vi "Read Sample Container.vi"(8 "error in (no error)":errorcluster, 11 "Preparation Line in":refnum<class "Preparation Line.lvclass">) -> (0 "error out":errorcluster, 1 "Sample":refnum<class "Sample.lvclass">, 2 "Container":T1, 3 "Preparation Line out":refnum<class "Preparation Line.lvclass">)   [LabVIEW 2015, in "cRIO-Carbondioxide.lvlib" / "CO2-Actor.lvlib" / "Preparation Line.lvclass"]
uses:
  Preparation Line.lvclass
  subs/Sample/Sample.lvclass
  Controls/Sample Container.ctl
  Preparation Line.lvclass/Preparation Line.ctl
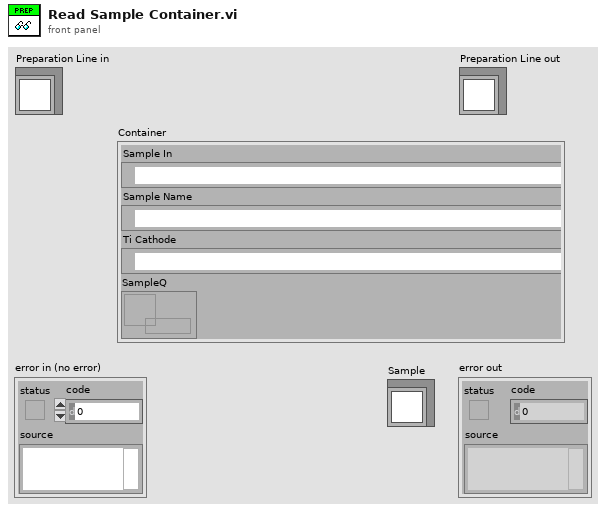
[diagram p1: front panel]
types:
  T1 = typedef "Sample Container.ctl" = cluster{"Sample In":refnum<k21>, "Sample Name":refnum<k21>, "Ti Cathode":refnum<k21>, "SampleQ":refnum<queue>}
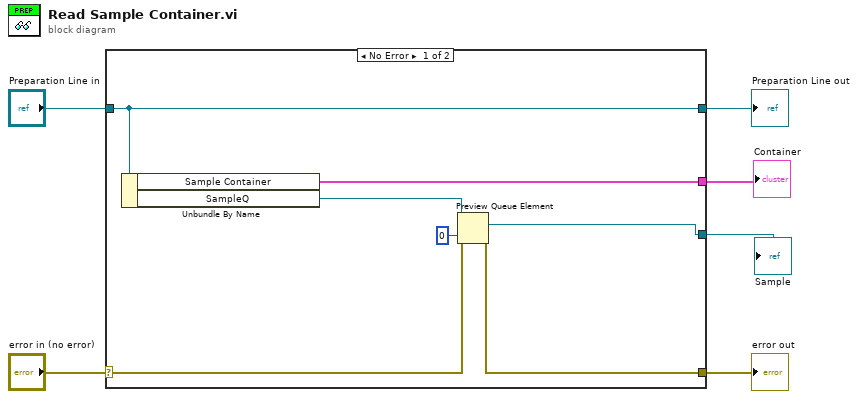
[diagram p0: block diagram]
diagram:
  n1 = case shown="No Error" "error in (no error)" {
    selector: "error in (no error)" -> [w8 w15]
    tunnel: [w7 w15] -> w4
    tunnel: [w13 w14] -> w3
    tunnel: "Preparation Line in" -> [w13 w14]
    tunnel: [w12 _] -> w2
    tunnel: [w9 _] -> w1
    frame No Error {
      n2 = Unbundle By Name(w13) -> ("Sample Container"=w12:T1, "SampleQ"=w10:refnum<queue>)
      n3 = Preview Queue Element(queue=w10, timeout in ms (-1)=0, error in (no error)=w8) -> (element=w9:refnum<class "Sample.lvclass">, error out=w7:errorcluster)  [unwired: 2 out]
    }
    frame Error {
    }
  }
  "error out" <- w4
  "Preparation Line out" <- w3
  "Container" <- w2
  "Sample" <- w1
